vi "Problem 14 - Longest Collatz sequence.vi"() -> ()   [LabVIEW 2021, in "Project Euler.lvlib"]
uses:
  Project Euler.lvlib
  Utilities/Numeric Utilities/Factors cluster.ctl
  Utilities/Named Timers/Named Timers.lvlib
  Utilities/Numeric Utilities/Numeric Utilities.lvlib
panel:
  out "T = U64 overflow;\nsequence has not ended":bool
  out "Factors out":T1[][](array[typedef])
  out "Array":bool[](array[boolean])
  in  "Offset":i32
  in  "Dev: stop early":bool
  out "n":u64
  out "Answer (number that generates longest sequence)":u64
  out "T = sanity check\nshould always be true":bool
  out "Longest Collatz sequence":u64[](array[numeric])
  out "longest no. of terms":i32
  out "Total execution time (ms)":u32
  # "Development\nControls or indicators that are useful for development or testing, but which are not outputs of the VI."
  # "Input\nInputs to the VI"
  # "Output\nOutputs of the VI"
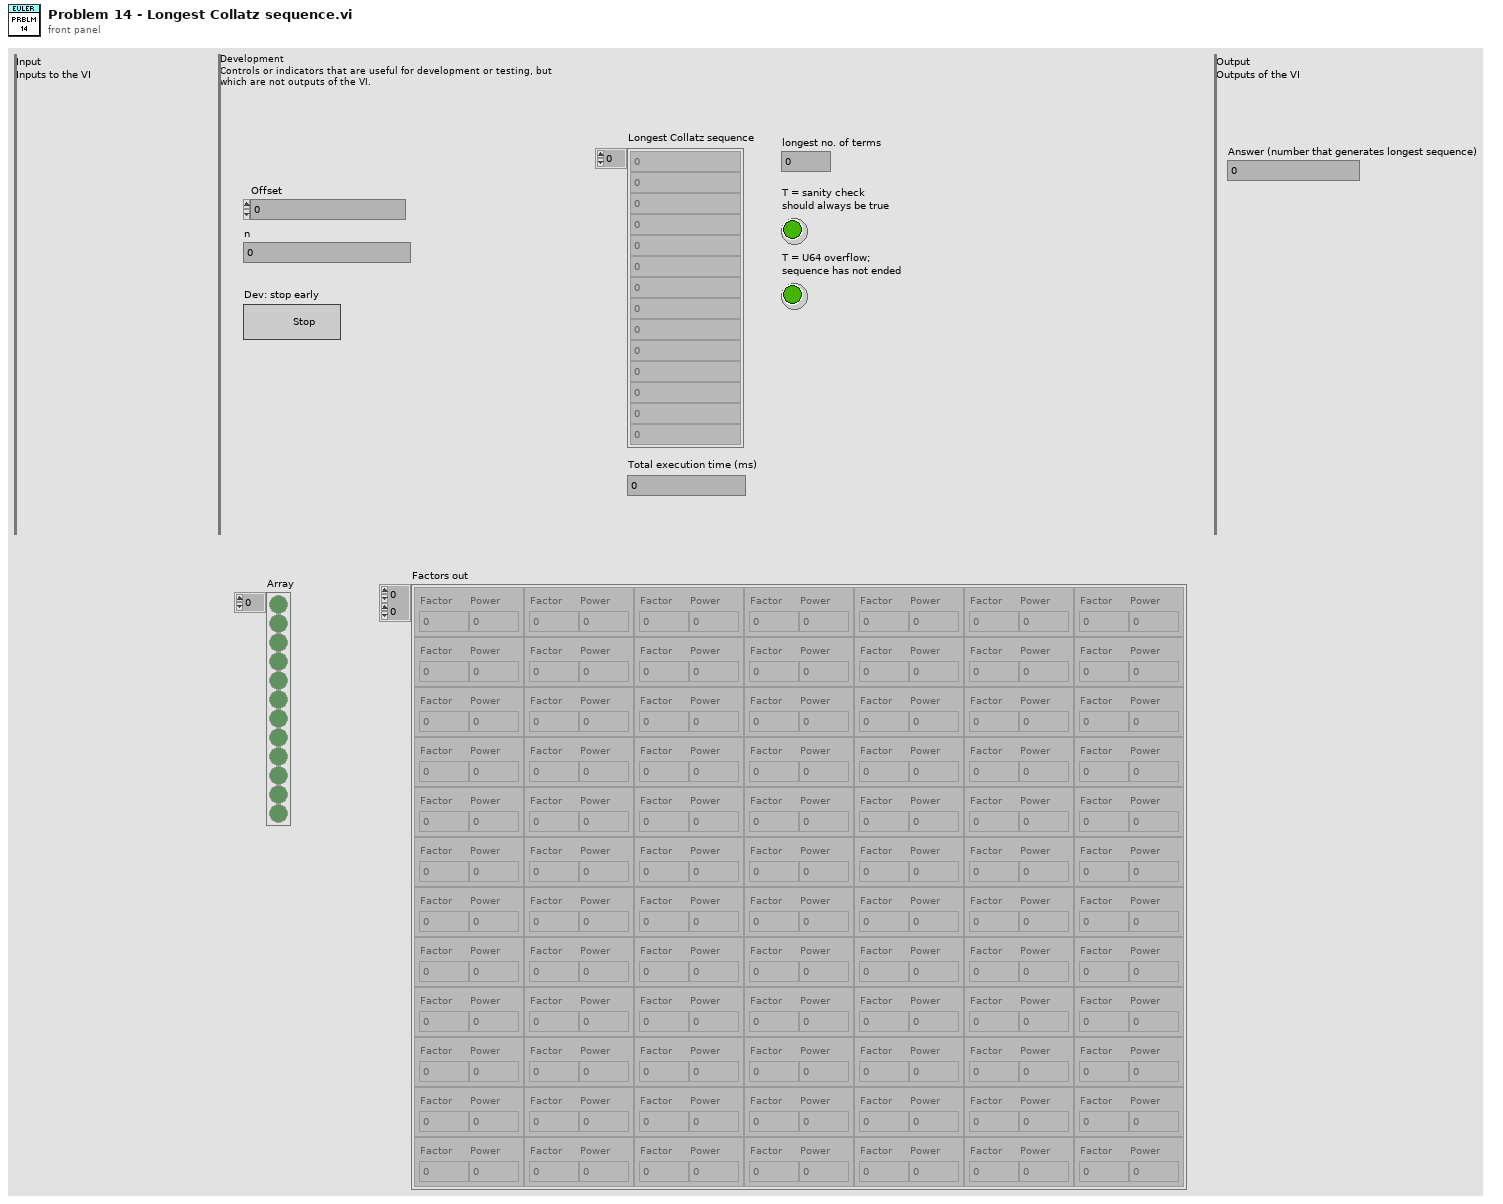
[diagram p1: front panel]
types:
  T1 = typedef "Numeric Utilities.lvlib/Factors cluster.ctl" = cluster{"Factor":i32, "Power":i32}
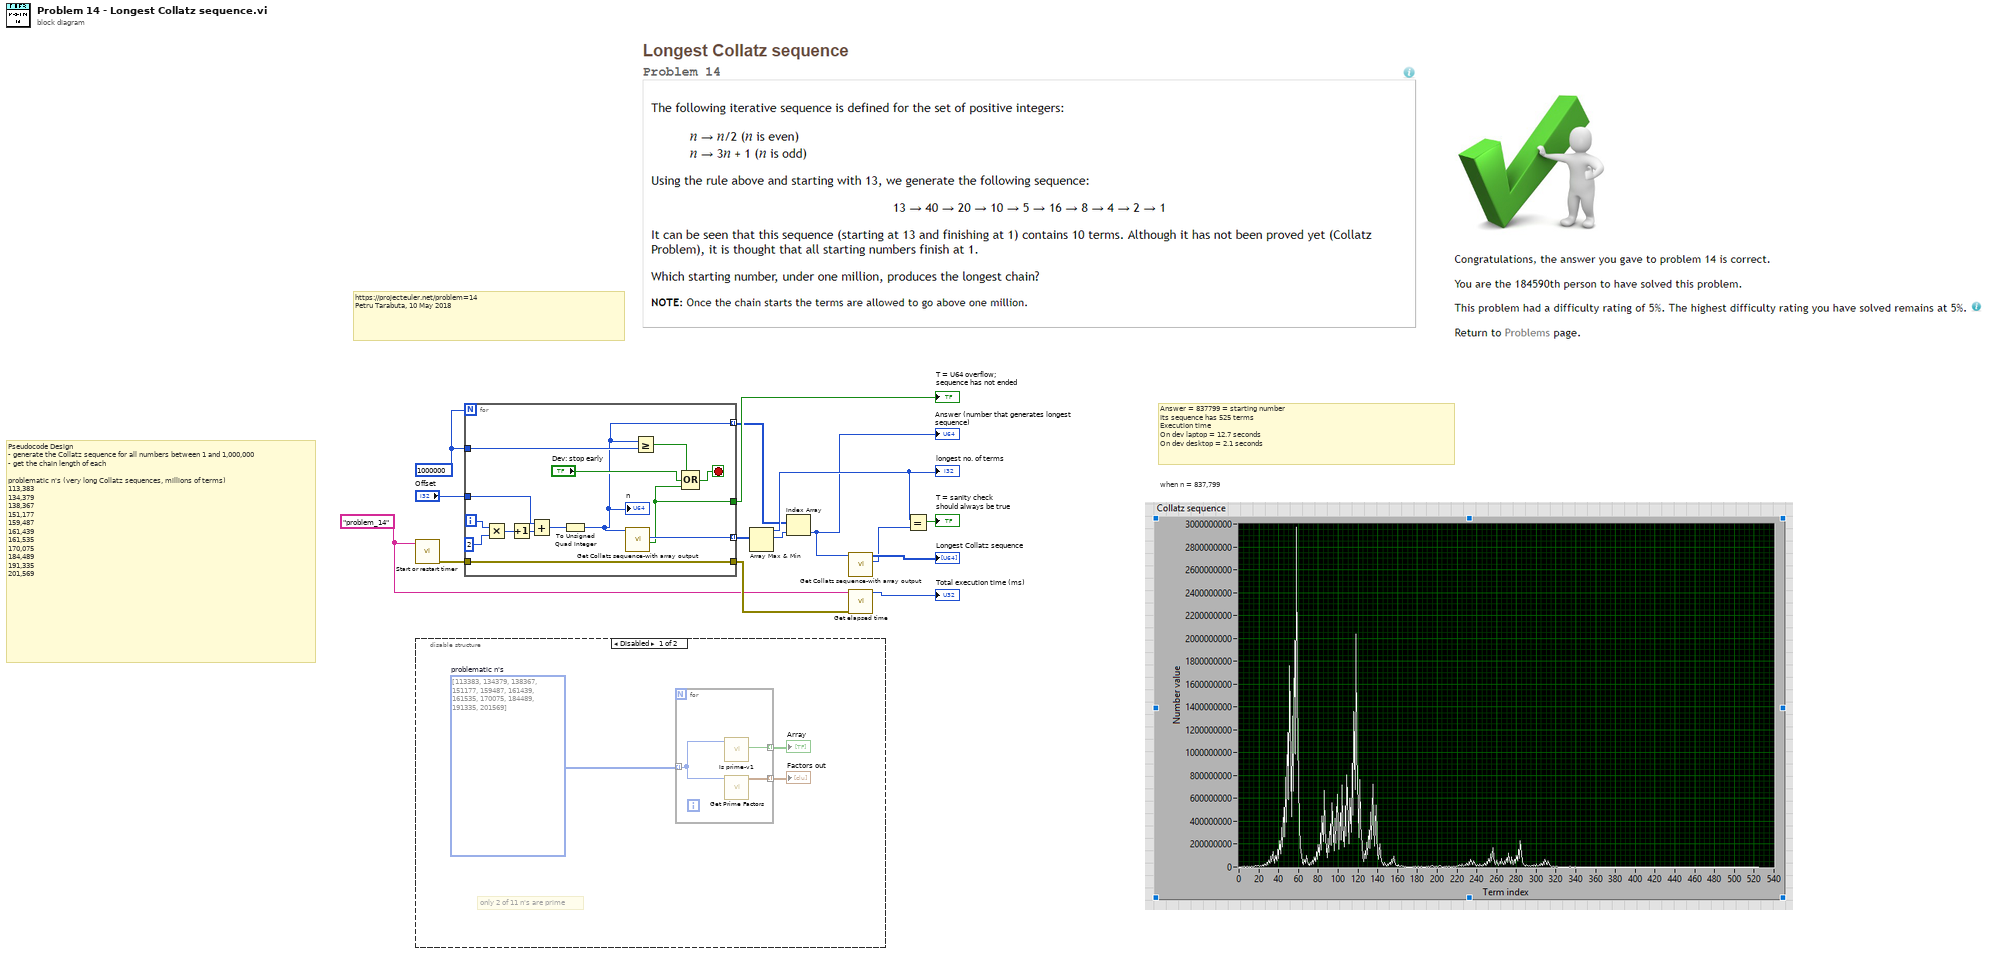
[diagram p0: block diagram]
diagram:
  w3 = 1000000
  w7 = "problem_14" ("Timer name")
  # "when n = 837,799"
  # "Pseudocode Design\n- generate the Collatz sequence for all numbers between 1 and 1,000,000\n- get the chain length of each\n\nproblematic n's (very long Collatz sequences, millions of terms)\n113,383\n134,379\n138,367\n151,177\n159,487\n161,439\n161,535\n170,075\n184,489\n191,335\n201,569"
  # "Answer = 837799 = starting number\nIts sequence has 525 terms\nExecution time\nOn dev laptop = 12.7 seconds\nOn dev desktop = 2.1 seconds"
  # "https://projecteuler.net/problem=14\nPetru Tarabuta, 10 May 2018"
  n1 = call "Start or restart timer.vi"("Timer name"=w7) -> ("error out"=w9:errorcluster)  [unwired: 10 in]
  n2 = disable-structure shown="Disabled" {
    frame Disabled {
      w18 = i32[] [113383, 134379, 138367, 151177, 159487, 161439, 161535, 170075, 184489, 191335, 201569]  # problematic n's
      # "only 2 of 11 n's are prime"
      n3 = for {
        tunnel: w18 -> [w20] mode=indexing
        tunnel: [w21] -> w17 mode=indexing
        tunnel: [w19] -> w16 mode=indexing
        n4 = call "Is prime-v1.vi"("x"=w20) -> ("T = x is prime"=w21:bool)  [unwired: 8 in, 2 out]
        n5 = call "Get Prime Factors.vi"("x"=w20) -> ("Factors out"=w19:T1[])  [unwired: 5 in, 5 out]
      }
      "Array" <- w17
      "Factors out" <- w16
    }
    frame Enabled {
    }
  }
  n6 = for {
    N: w3 -> [_]
    tunnel: [w34] -> w14 mode=indexing
    tunnel: w9 -> [w33]
    tunnel: [w33] -> w8
    tunnel: "Offset" -> [w31]
    tunnel: [w28] -> w4
    tunnel: w3 -> [w27]
    tunnel: [w22] -> w2 mode=indexing
    i -> [w25]
    stop <- w29 stop-if-true
    n7 = Multiply(x=w25, y=2) -> (x*y=w23:i32)
    n8 = Increment(x=w23) -> (x+1=w35:i32)
    n9 = Add(x=w31, y=w35) -> (x+y=w32:i32)
    n10 = To Unsigned Quad Integer(1:w32) -> (0:w22:u64)
    "n" <- w22
    n11 = call "Get Collatz sequence-with array output.vi"("n"=w22) -> ("T = U64 overflow\nsequence has not ended"=w28:bool, "no. of elements (chain length)"=w34:i32)  [unwired: 7 in, 2 out]
    n12 = Greater Or Equal?(x=w22, y=w27) -> (x >= y?=w26:bool)
    n13 = Compound Arithmetic op=OR(w26, "Dev: stop early", w28) -> (w29:bool)
  }
  "T = U64 overflow;\nsequence has not ended" <- w4
  n14 = Array Max & Min(array=w14) -> (max value=w12:i32, max index (indices)=w1:i32)  [unwired: 2 out]
  "longest no. of terms" <- w12
  n15 = Index Array(array=w2, index=w1) -> (element=w5:u64)
  "Answer (number that generates longest sequence)" <- w5
  n16 = call "Get Collatz sequence-with array output.vi"("n"=w5) -> ("no. of elements (chain length)"=w11:i32, "Collatz sequence of n"=→"Longest Collatz sequence":u64[])  [unwired: 7 in, 2 out]
  n17 = call "Get elapsed time.vi"("error in (no error)"=w8, "Timer name"=w7) -> ("Elapsed time (ms)"=→"Total execution time (ms)":u32)  [unwired: 6 in, 3 out]
  n18 = Equal?(x=w12, y=w11) -> (x = y?=→"T = sanity check\nshould always be true":bool)
